vi "TestFriction.vi"(9 "边界配置":T2={"x1"=-90.0, "x2"=90.0, "lower"=4.9, "upper"=5.1}, 11 "原始曲线":cluster{"X":sgl[], "Y":sgl[]}) -> (1 "运算值":T1, 3 "曲线数组":cluster{"X":dbl[], "Y":dbl[]}[](array[cluster]))   [LabVIEW 2018]
panel:
  out "XY图 2":cluster{"右角度":dbl[], "右扭矩":dbl[]}[](graph)
  # "如果边界upper设定为负数，则max与min交换数据！"
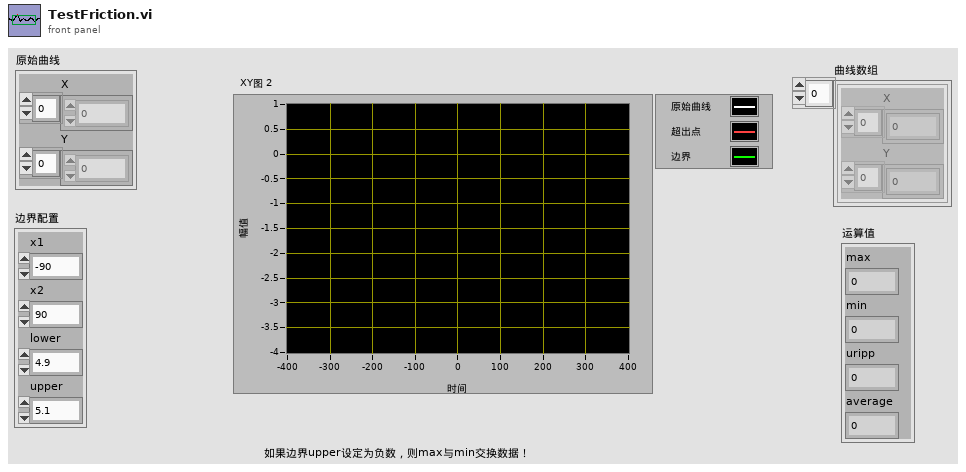
[diagram p1: front panel]
types:
  T1 = cluster{"max":dbl, "min":dbl, "uripp":dbl, "average":dbl}
  T2 = cluster{"x1":dbl, "x2":dbl, "lower":dbl, "upper":dbl}
  T3 = cluster{"x1":dbl, "lower":dbl, "upper":dbl, "x2":dbl, "lower":dbl, "upper":dbl}
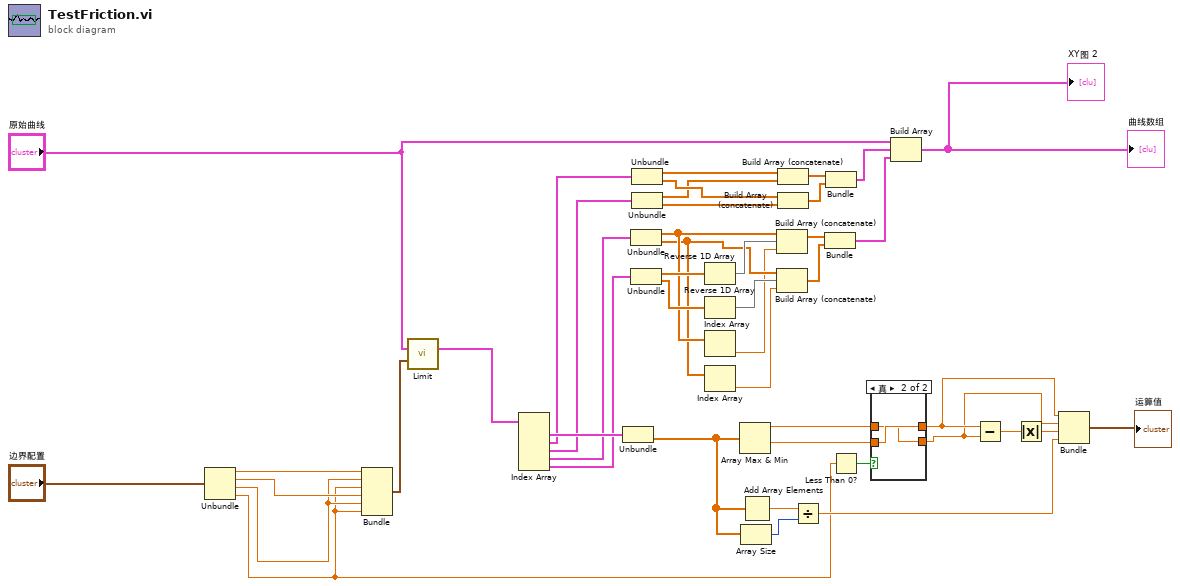
[diagram p0: block diagram]
diagram:
  n1 = Unbundle("边界配置") -> ("x1"=w44:dbl, "x2"=w43:dbl, "lower"=w42:dbl, "upper"=w27:dbl)
  n2 = Bundle("x1"=w44, "lower"=w42, "upper"=w27, "x2"=w43, "lower"=w42, "upper"=w27) -> (w41:T3)  [unwired: 1 in]
  n3 = call "Limit.vi"("XY_in"="原始曲线", "边界配置"=w41) -> ("XY_out"=w40:cluster{dbl[], dbl[]}[])  [unwired: 12 in, 1 out]
  n4 = Index Array(array=w40) -> (element #1=w39:cluster{dbl[], dbl[]}, element #2=w14:cluster{dbl[], dbl[]}, element #3=w13:cluster{dbl[], dbl[]}, element #4=w22:cluster{dbl[], dbl[]}, element #5=w21:cluster{dbl[], dbl[]})  [unwired: 5 in]
  n5 = Unbundle(w39) -> (w36:dbl[])  [unwired: 1 out]
  n6 = Unbundle(w22) -> (w5:dbl[], w4:dbl[])
  n7 = Unbundle(w21) -> (w9:dbl[], w7:dbl[])
  n8 = Unbundle(w14) -> (w15:dbl[], w17:dbl[])
  n9 = Unbundle(w13) -> (w16:dbl[], w18:dbl[])
  n10 = Reverse 1D Array(array=w9) -> (reversed array=w8:dbl[])
  n11 = Reverse 1D Array(array=w7) -> (reversed array=w6:dbl[])
  n12 = Index Array(array=w5) -> (element=w3:dbl)  [unwired: 1 in]
  n13 = Index Array(array=w4) -> (element=w2:dbl)  [unwired: 1 in]
  n14 = Array Max & Min(array=w36) -> (max value=w35:dbl, min value=w34:dbl)  [unwired: 2 out]
  n15 = Array Size(array=w36) -> (size(s)=w38:i32)
  n16 = Add Array Elements(numeric array=w36) -> (sum=w37:dbl)
  n17 = Build Array (concatenate)(w5, w8, w3) -> (w24:dbl[])
  n18 = Build Array (concatenate)(w4, w6, w2) -> (w23:dbl[])
  n19 = Build Array (concatenate)(w15, w16) -> (w19:dbl[])
  n20 = Build Array (concatenate)(w17, w18) -> (w20:dbl[])
  n21 = Divide(x=w37, y=w38) -> (x/y=w33:dbl)
  n22 = Bundle(w24, w23) -> (w11:cluster{dbl[], dbl[]})  [unwired: 1 in]
  n23 = Bundle(w19, w20) -> (w12:cluster{dbl[], dbl[]})  [unwired: 1 in]
  n24 = Less Than 0?(x=w27) -> (x < 0?=w32:bool)
  n25 = case shown="真" w32 {
    tunnel: w35 -> [w46 w47]
    tunnel: [w46 w48] -> w31
    tunnel: w34 -> [w45 w48]
    tunnel: [w45 w47] -> w30
    frame False {
    }
    frame True {
    }
  }
  n26 = Build Array("原始曲线", w12, w11) -> (→"XY图 2" →"曲线数组":cluster{"X":dbl[], "Y":dbl[]}[])
  n27 = Subtract(x=w31, y=w30) -> (x-y=w26:dbl)
  n28 = Absolute Value(x=w26) -> (abs(x)=w25:dbl)
  n29 = Bundle(w31, w30, w25, w33) -> (→"运算值":cluster{dbl, dbl, dbl, dbl})  [unwired: 1 in]
